vi "Control.vi"() -> ()   [LabVIEW 2018, in "BigSkyControl.lvlib"]
uses:
  BigSkyControl.lvlib
  VISAGlobal.vi
panel:
  out "Resonse History":string
  in  "Command (no > or \\r\\n)":string
  in  "Send Command":bool
  in  "Frequency[Hz]":dbl=7.0 min=0.01 max=56.0 step=0.01 format="%.2g"
  in  "Query Frequency":bool
  in  "Set Frequency":bool
  in  "Query Temperature":bool
  in  "Query Shutter":bool
  in  "Single QSwitch":bool
  in  "Stop QSwitch":bool
  in  "Start QSwitch":bool
  in  "Query Voltage":bool
  in  "Set Voltage":bool
  in  "Stop":bool
  out "Voltage Reported":dbl format="%_4f"
  in  "Voltage[V]":dbl(slide)=700.0 min=700.0 max=950.0 step=5.0 scale=700.0..950.0
  in  "Stop Lamps":bool
  in  "Warmup Lamps":bool
  out "Response":string
  in  "Close shutter":bool
  in  "Open shutter":bool
  in  "VISA resource name":refnum<visa-resource-name>="COM1"
  # "System"
  # "Lamp Control"
  # "Q-Switch Control"
  # "Shutter Control"
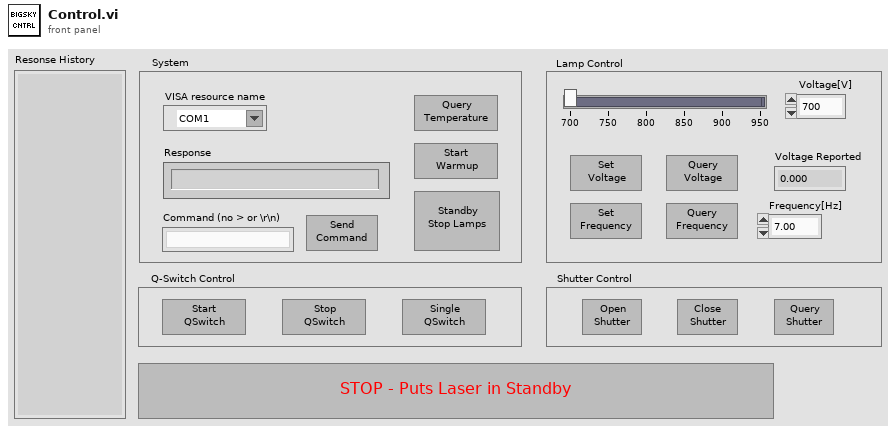
[diagram p1: front panel]
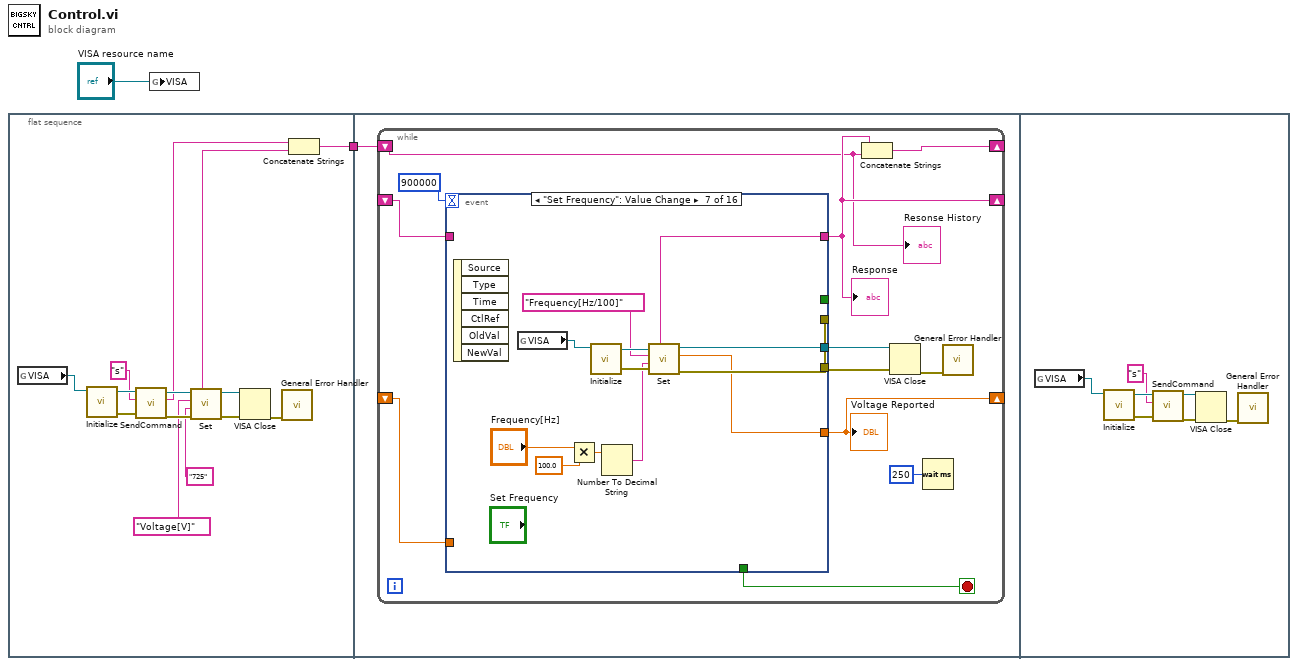
[diagram p0: block diagram]
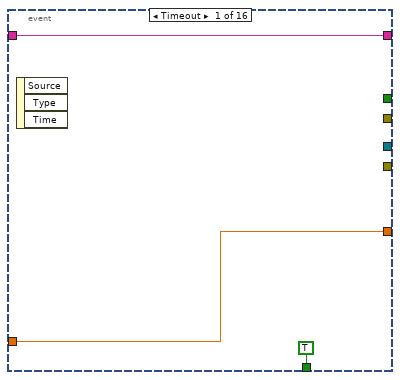
[diagram p2: hidden frame]
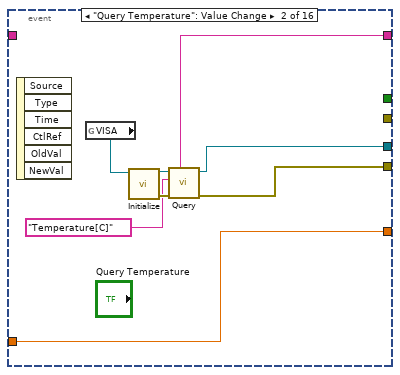
[diagram p3: hidden frame]
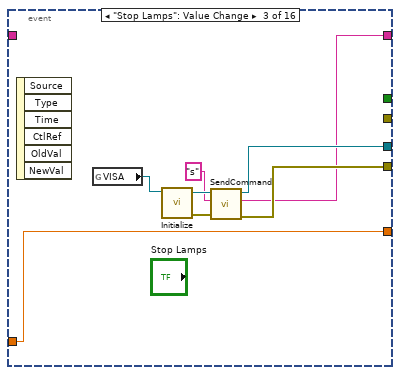
[diagram p4: hidden frame]
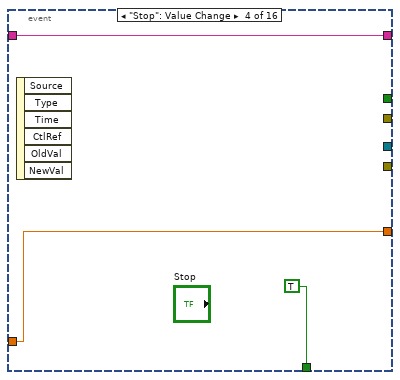
[diagram p5: hidden frame]
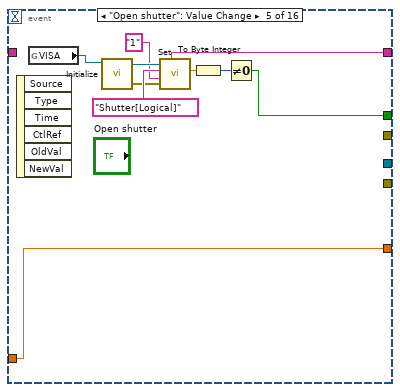
[diagram p6: hidden frame]
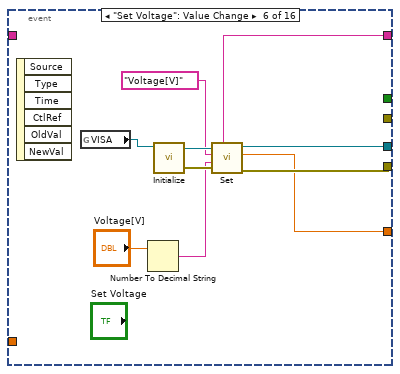
[diagram p7: hidden frame]
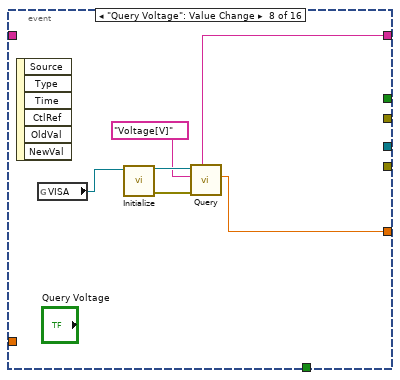
[diagram p8: hidden frame]
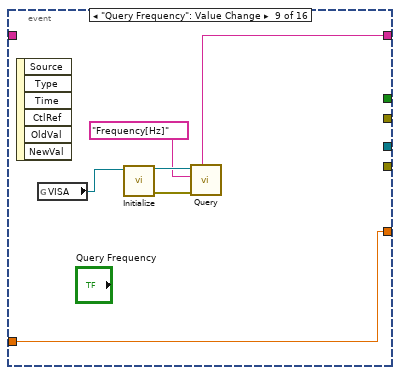
[diagram p9: hidden frame]
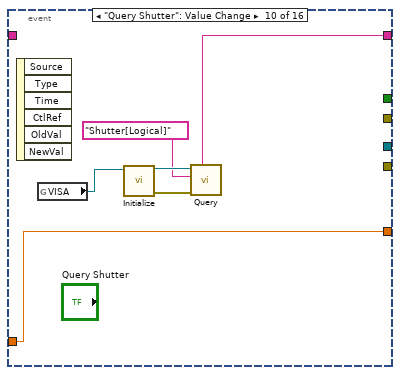
[diagram p10: hidden frame]
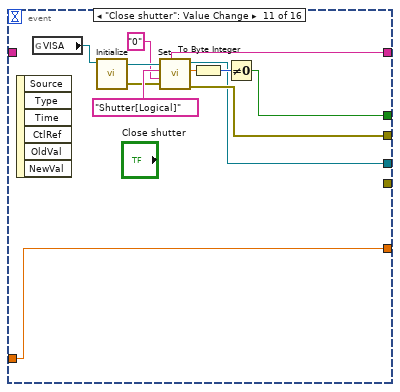
[diagram p11: hidden frame]
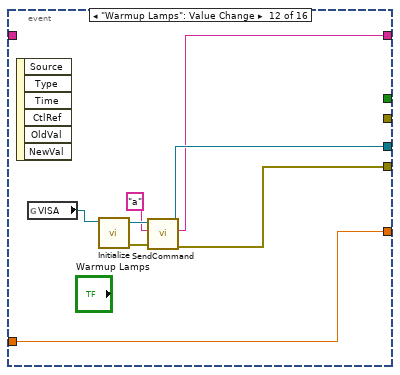
[diagram p12: hidden frame]
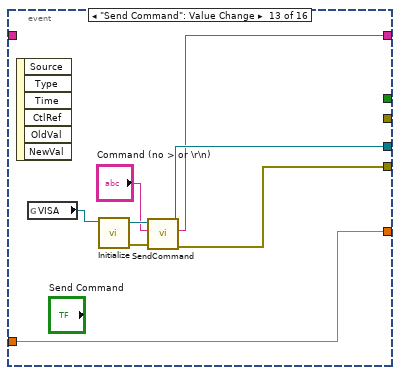
[diagram p13: hidden frame]
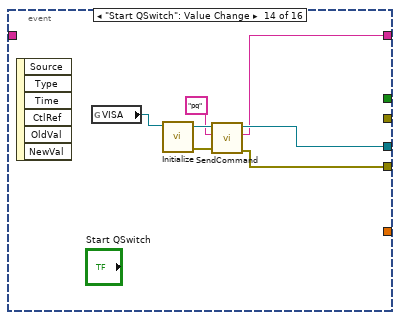
[diagram p14: hidden frame]
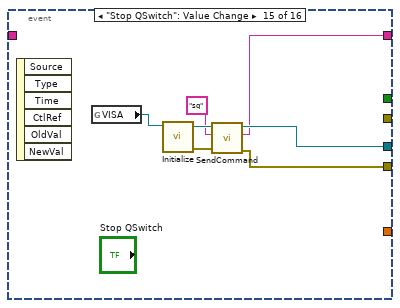
[diagram p15: hidden frame]
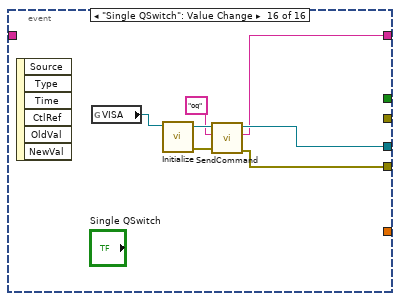
[diagram p16: hidden frame]
diagram:
  n1 = flat-sequence {
    tunnel: [w3] -> w1
    tunnel: w1 -> [w17]
    frame #0 {
      n2 = global read "VISAGlobal.vi" "VISA"() -> (w13:refnum<visa-resource-name>)
      n3 = call "Initialize.vi"("VISA resource name"=w13) -> ("error out"=w15:errorcluster, "VISA resource name out"=w16:refnum<visa-resource-name>)  [unwired: 7 in]
      n4 = call "SendCommand.vi"("error"=w15, "write buffer (don't include >\\r\\n)"="s" ("write buffer (don't include >\\r\\n)"), "VISA resource name"=w16) -> ("error out"=w10:errorcluster, "Response"=w5:string, "VISA resource name out"=w11:refnum<visa-resource-name>)  [unwired: 6 in]
      n5 = call "Set.vi"("error"=w10, "Input Command String"="725", "Quantity"="Voltage[V]", "VISA resource name"=w11) -> ("error out"=w7:errorcluster, "VISA resource name out"=w8:refnum<visa-resource-name>, "Response"=w6:string)  [unwired: 2 in, 1 out]
      n6 = VISA Close(VISA resource name=w8, error in (no error)=w7) -> (error out=w12:errorcluster)
      n7 = call <vilib>:"General Error Handler.vi"("error in (no error)"=w12) -> ()  [unwired: 10 in, 5 out]
      n8 = Concatenate Strings(w5, w6) -> (w3:string)
    }
    frame #1 {
      n9 = while {
        shift-right: [w19] -> _
        shift-left: _ -> [w23]
        shift-right: [w22] -> _
        shift-left: _ -> [w21]
        shift-right: [w20] -> _
        shift-left: w17 -> [w18]
        stop <- w25 stop-if-true
        n10 = event shown="[6] \"Set Frequency\": Value Change" {
          selector: _ -> [_ _ _ _ _ _ _ _ _ _ _ _ _ _ _ _]
          dyn-events: _ -> [_ _ _ _ _ _ _ _ _ _ _ _ _ _ _ _]
          timeout: 900000 -> [_ _ _ _ _ _ _ _ _ _ _ _ _ _ _ _]
          tunnel: [w32 w39 w42 w50 w58 w68 w80 w84 w91 w97 w110 w115 w124 w130 w137 w144] -> w19
          tunnel: [_ _ _ _ w55 _ _ _ _ _ w107 _ _ _ _ _] -> _
          tunnel: [_ _ _ _ _ _ _ _ _ _ w105 _ _ _ _ _] -> w29
          tunnel: [_ w38 w44 _ _ w64 w78 _ _ _ w104 w117 w126 w131 w138 w145] -> w28
          tunnel: [_ w37 w43 _ _ w63 w77 _ _ _ _ w116 w125 w132 w139 w146] -> _
          tunnel: [TRUE _ _ TRUE _ _ _ _ _ _ _ _ _ _ _ _] -> w25
          tunnel: [w31 w40 w41 w49 w52 w62 w76 w85 w90 w96 w102 w114 w123 _ _ _] -> w22
          tunnel: w23 -> [w32 _ _ w50 _ _ _ _ _ _ _ _ _ _ _ _]
          tunnel: w21 -> [w31 w40 w41 w49 w52 _ _ _ w90 w96 w102 w114 w123 _ _ _]
          event Timeout {
            n11 = event-data() -> ()  [unwired: 1 in, 3 out]
          }
          event "Query Temperature": Value Change {
            n12 = event-data() -> ()  [unwired: 1 in, 6 out]
            n13 = global read "VISAGlobal.vi" "VISA"() -> (w34:refnum<visa-resource-name>)
            n14 = call "Initialize.vi"("VISA resource name"=w34) -> ("error out"=w35:errorcluster, "VISA resource name out"=w36:refnum<visa-resource-name>)  [unwired: 7 in]
            n15 = call "Query.vi"("error"=w35, "Quantity"="Temperature[C]", "VISA resource name"=w36) -> ("error out"=w37:errorcluster, "VISA resource name out"=w38:refnum<visa-resource-name>, "Response"=w39:string)  [unwired: 3 in, 1 out]
          }
          event "Stop Lamps": Value Change {
            n16 = event-data() -> ()  [unwired: 1 in, 6 out]
            n17 = global read "VISAGlobal.vi" "VISA"() -> (w45:refnum<visa-resource-name>)
            n18 = call "Initialize.vi"("VISA resource name"=w45) -> ("error out"=w47:errorcluster, "VISA resource name out"=w48:refnum<visa-resource-name>)  [unwired: 7 in]
            n19 = call "SendCommand.vi"("error"=w47, "write buffer (don't include >\\r\\n)"="s" ("write buffer (don't include >\\r\\n)"), "VISA resource name"=w48) -> ("error out"=w43:errorcluster, "Response"=w42:string, "VISA resource name out"=w44:refnum<visa-resource-name>)  [unwired: 6 in]
          }
          event "Stop": Value Change {
            n20 = event-data() -> ()  [unwired: 1 in, 6 out]
          }
          event "Open shutter": Value Change {
            n21 = event-data() -> ()  [unwired: 1 in, 6 out]
            n22 = global read "VISAGlobal.vi" "VISA"() -> (w53:refnum<visa-resource-name>)
            n23 = call "Initialize.vi"("VISA resource name"=w53) -> ("error out"=w59:errorcluster, "VISA resource name out"=w60:refnum<visa-resource-name>)  [unwired: 7 in]
            n24 = call "Set.vi"("error"=w59, "Input Command String"="1", "Quantity"="Shutter[Logical]", "VISA resource name"=w60) -> ("Returned"=w57:dbl, "Response"=w58:string)  [unwired: 2 in, 2 out]
            n25 = To Byte Integer(number=w57) -> (8bit integer=w56:i8)
            n26 = Not Equal To 0?(x=w56) -> (x != 0?=w55:bool)
          }
          event "Set Voltage": Value Change {
            n27 = event-data() -> ()  [unwired: 1 in, 6 out]
            n28 = global read "VISAGlobal.vi" "VISA"() -> (w69:refnum<visa-resource-name>)
            n29 = Number To Decimal String(number="Voltage[V]") -> (decimal integer string=w65:string)  [unwired: 1 in]
            n30 = call "Initialize.vi"("VISA resource name"=w69) -> ("error out"=w70:errorcluster, "VISA resource name out"=w71:refnum<visa-resource-name>)  [unwired: 7 in]
            n31 = call "Set.vi"("error"=w70, "Input Command String"=w65, "Quantity"="Voltage[V]", "VISA resource name"=w71) -> ("error out"=w63:errorcluster, "Returned"=w62:dbl, "VISA resource name out"=w64:refnum<visa-resource-name>, "Response"=w68:string)  [unwired: 2 in]
          }
          event "Set Frequency": Value Change {
            n32 = event-data() -> ()  [unwired: 1 in, 6 out]
            n33 = global read "VISAGlobal.vi" "VISA"() -> (w81:refnum<visa-resource-name>)
            n34 = Multiply(x="Frequency[Hz]", y=100.0) -> (x*y=w73:dbl)
            n35 = call "Initialize.vi"("VISA resource name"=w81) -> ("error out"=w82:errorcluster, "VISA resource name out"=w83:refnum<visa-resource-name>)  [unwired: 7 in]
            n36 = Number To Decimal String(number=w73) -> (decimal integer string=w79:string)  [unwired: 1 in]
            n37 = call "Set.vi"("error"=w82, "Input Command String"=w79, "Quantity"="Frequency[Hz/100]", "VISA resource name"=w83) -> ("error out"=w77:errorcluster, "Returned"=w76:dbl, "VISA resource name out"=w78:refnum<visa-resource-name>, "Response"=w80:string)  [unwired: 2 in]
          }
          event "Query Voltage": Value Change {
            n38 = event-data() -> ()  [unwired: 1 in, 6 out]
            n39 = global read "VISAGlobal.vi" "VISA"() -> (w87:refnum<visa-resource-name>)
            n40 = call "Initialize.vi"("VISA resource name"=w87) -> ("error out"=w88:errorcluster, "VISA resource name out"=w89:refnum<visa-resource-name>)  [unwired: 7 in]
            n41 = call "Query.vi"("error"=w88, "Quantity"="Voltage[V]", "VISA resource name"=w89) -> ("Value"=w85:dbl, "Response"=w84:string)  [unwired: 3 in, 2 out]
          }
          event "Query Frequency": Value Change {
            n42 = event-data() -> ()  [unwired: 1 in, 6 out]
            n43 = global read "VISAGlobal.vi" "VISA"() -> (w93:refnum<visa-resource-name>)
            n44 = call "Initialize.vi"("VISA resource name"=w93) -> ("error out"=w94:errorcluster, "VISA resource name out"=w95:refnum<visa-resource-name>)  [unwired: 7 in]
            n45 = call "Query.vi"("error"=w94, "Quantity"="Frequency[Hz]", "VISA resource name"=w95) -> ("Response"=w91:string)  [unwired: 3 in, 3 out]
          }
          event "Query Shutter": Value Change {
            n46 = event-data() -> ()  [unwired: 1 in, 6 out]
            n47 = global read "VISAGlobal.vi" "VISA"() -> (w99:refnum<visa-resource-name>)
            n48 = call "Initialize.vi"("VISA resource name"=w99) -> ("error out"=w100:errorcluster, "VISA resource name out"=w101:refnum<visa-resource-name>)  [unwired: 7 in]
            n49 = call "Query.vi"("error"=w100, "Quantity"="Shutter[Logical]", "VISA resource name"=w101) -> ("Response"=w97:string)  [unwired: 3 in, 3 out]
          }
          event "Close shutter": Value Change {
            n50 = event-data() -> ()  [unwired: 1 in, 6 out]
            n51 = global read "VISAGlobal.vi" "VISA"() -> (w103:refnum<visa-resource-name>)
            n52 = call "Initialize.vi"("VISA resource name"=w103) -> ("error out"=w111:errorcluster, "VISA resource name out"=w112:refnum<visa-resource-name>)  [unwired: 7 in]
            n53 = call "Set.vi"("error"=w111, "Input Command String"="0", "Quantity"="Shutter[Logical]", "VISA resource name"=w112) -> ("error out"=w105:errorcluster, "Returned"=w109:dbl, "VISA resource name out"=w104:refnum<visa-resource-name>, "Response"=w110:string)  [unwired: 2 in]
            n54 = To Byte Integer(number=w109) -> (8bit integer=w108:i8)
            n55 = Not Equal To 0?(x=w108) -> (x != 0?=w107:bool)
          }
          event "Warmup Lamps": Value Change {
            n56 = event-data() -> ()  [unwired: 1 in, 6 out]
            n57 = global read "VISAGlobal.vi" "VISA"() -> (w118:refnum<visa-resource-name>)
            n58 = call "Initialize.vi"("VISA resource name"=w118) -> ("error out"=w120:errorcluster, "VISA resource name out"=w121:refnum<visa-resource-name>)  [unwired: 7 in]
            n59 = call "SendCommand.vi"("error"=w120, "write buffer (don't include >\\r\\n)"="a" ("write buffer (don't include >\\r\\n)"), "VISA resource name"=w121) -> ("error out"=w116:errorcluster, "Response"=w115:string, "VISA resource name out"=w117:refnum<visa-resource-name>)  [unwired: 6 in]
          }
          event "Send Command": Value Change {
            n60 = event-data() -> ()  [unwired: 1 in, 6 out]
            n61 = global read "VISAGlobal.vi" "VISA"() -> (w127:refnum<visa-resource-name>)
            n62 = call "Initialize.vi"("VISA resource name"=w127) -> ("error out"=w128:errorcluster, "VISA resource name out"=w129:refnum<visa-resource-name>)  [unwired: 7 in]
            n63 = call "SendCommand.vi"("error"=w128, "write buffer (don't include >\\r\\n)"="Command (no > or \\r\\n)", "VISA resource name"=w129) -> ("error out"=w125:errorcluster, "Response"=w124:string, "VISA resource name out"=w126:refnum<visa-resource-name>)  [unwired: 6 in]
          }
          event "Start QSwitch": Value Change {
            n64 = event-data() -> ()  [unwired: 1 in, 6 out]
            n65 = global read "VISAGlobal.vi" "VISA"() -> (w133:refnum<visa-resource-name>)
            n66 = call "Initialize.vi"("VISA resource name"=w133) -> ("error out"=w135:errorcluster, "VISA resource name out"=w136:refnum<visa-resource-name>)  [unwired: 7 in]
            n67 = call "SendCommand.vi"("error"=w135, "write buffer (don't include >\\r\\n)"="pq" ("write buffer (don't include >\\r\\n)"), "VISA resource name"=w136) -> ("error out"=w132:errorcluster, "Response"=w130:string, "VISA resource name out"=w131:refnum<visa-resource-name>)  [unwired: 6 in]
          }
          event "Stop QSwitch": Value Change {
            n68 = event-data() -> ()  [unwired: 1 in, 6 out]
            n69 = global read "VISAGlobal.vi" "VISA"() -> (w140:refnum<visa-resource-name>)
            n70 = call "Initialize.vi"("VISA resource name"=w140) -> ("error out"=w142:errorcluster, "VISA resource name out"=w143:refnum<visa-resource-name>)  [unwired: 7 in]
            n71 = call "SendCommand.vi"("error"=w142, "write buffer (don't include >\\r\\n)"="sq" ("write buffer (don't include >\\r\\n)"), "VISA resource name"=w143) -> ("error out"=w139:errorcluster, "Response"=w137:string, "VISA resource name out"=w138:refnum<visa-resource-name>)  [unwired: 6 in]
          }
          event "Single QSwitch": Value Change {
            n72 = event-data() -> ()  [unwired: 1 in, 6 out]
            n73 = global read "VISAGlobal.vi" "VISA"() -> (w147:refnum<visa-resource-name>)
            n74 = call "Initialize.vi"("VISA resource name"=w147) -> ("error out"=w149:errorcluster, "VISA resource name out"=w150:refnum<visa-resource-name>)  [unwired: 7 in]
            n75 = call "SendCommand.vi"("error"=w149, "write buffer (don't include >\\r\\n)"="oq" ("write buffer (don't include >\\r\\n)"), "VISA resource name"=w150) -> ("error out"=w146:errorcluster, "Response"=w144:string, "VISA resource name out"=w145:refnum<visa-resource-name>)  [unwired: 6 in]
          }
        }
        "Response" <- w19
        "Voltage Reported" <- w22
        n76 = Concatenate Strings(w19, w18) -> (w20:string)
        n77 = VISA Close(VISA resource name=w28, error in (no error)=w29) -> (error out=w27:errorcluster)
        n78 = Wait (ms)(milliseconds to wait=u32 250) -> ()  [unwired: 1 out]
        n79 = call <vilib>:"General Error Handler.vi"("error in (no error)"=w27) -> ()  [unwired: 10 in, 5 out]
        "Resonse History" <- w18
      }
    }
    frame #2 {
      n80 = global read "VISAGlobal.vi" "VISA"() -> (w154:refnum<visa-resource-name>)
      n81 = call "Initialize.vi"("VISA resource name"=w154) -> ("error out"=w156:errorcluster, "VISA resource name out"=w157:refnum<visa-resource-name>)  [unwired: 7 in]
      n82 = call "SendCommand.vi"("error"=w156, "write buffer (don't include >\\r\\n)"="s" ("write buffer (don't include >\\r\\n)"), "VISA resource name"=w157) -> ("error out"=w151:errorcluster, "VISA resource name out"=w152:refnum<visa-resource-name>)  [unwired: 6 in, 1 out]
      n83 = VISA Close(VISA resource name=w152, error in (no error)=w151) -> (error out=w153:errorcluster)
      n84 = call <vilib>:"General Error Handler.vi"("error in (no error)"=w153) -> ()  [unwired: 10 in, 5 out]
    }
  }
  n85 = global write "VISAGlobal.vi" "VISA"("VISA resource name") -> ()
